vi "testing_camera_settings.vi"() -> ()   [LabVIEW 2015]
panel:
  out "Expected Rate":dbl
  out "millisecond timer value":u32
  out "imaq error":errorcluster
  out "dcam error":errorcluster {"code" format="%.0x"}
  out "Acquiring Frames":bool
  out "Frames Recorded":i32
  out "Display":T1(plugin-control)
  out "Current Stim Frames":i32
  out "H Width":i32
  out "V Width":i32
  out "Exposure":dbl
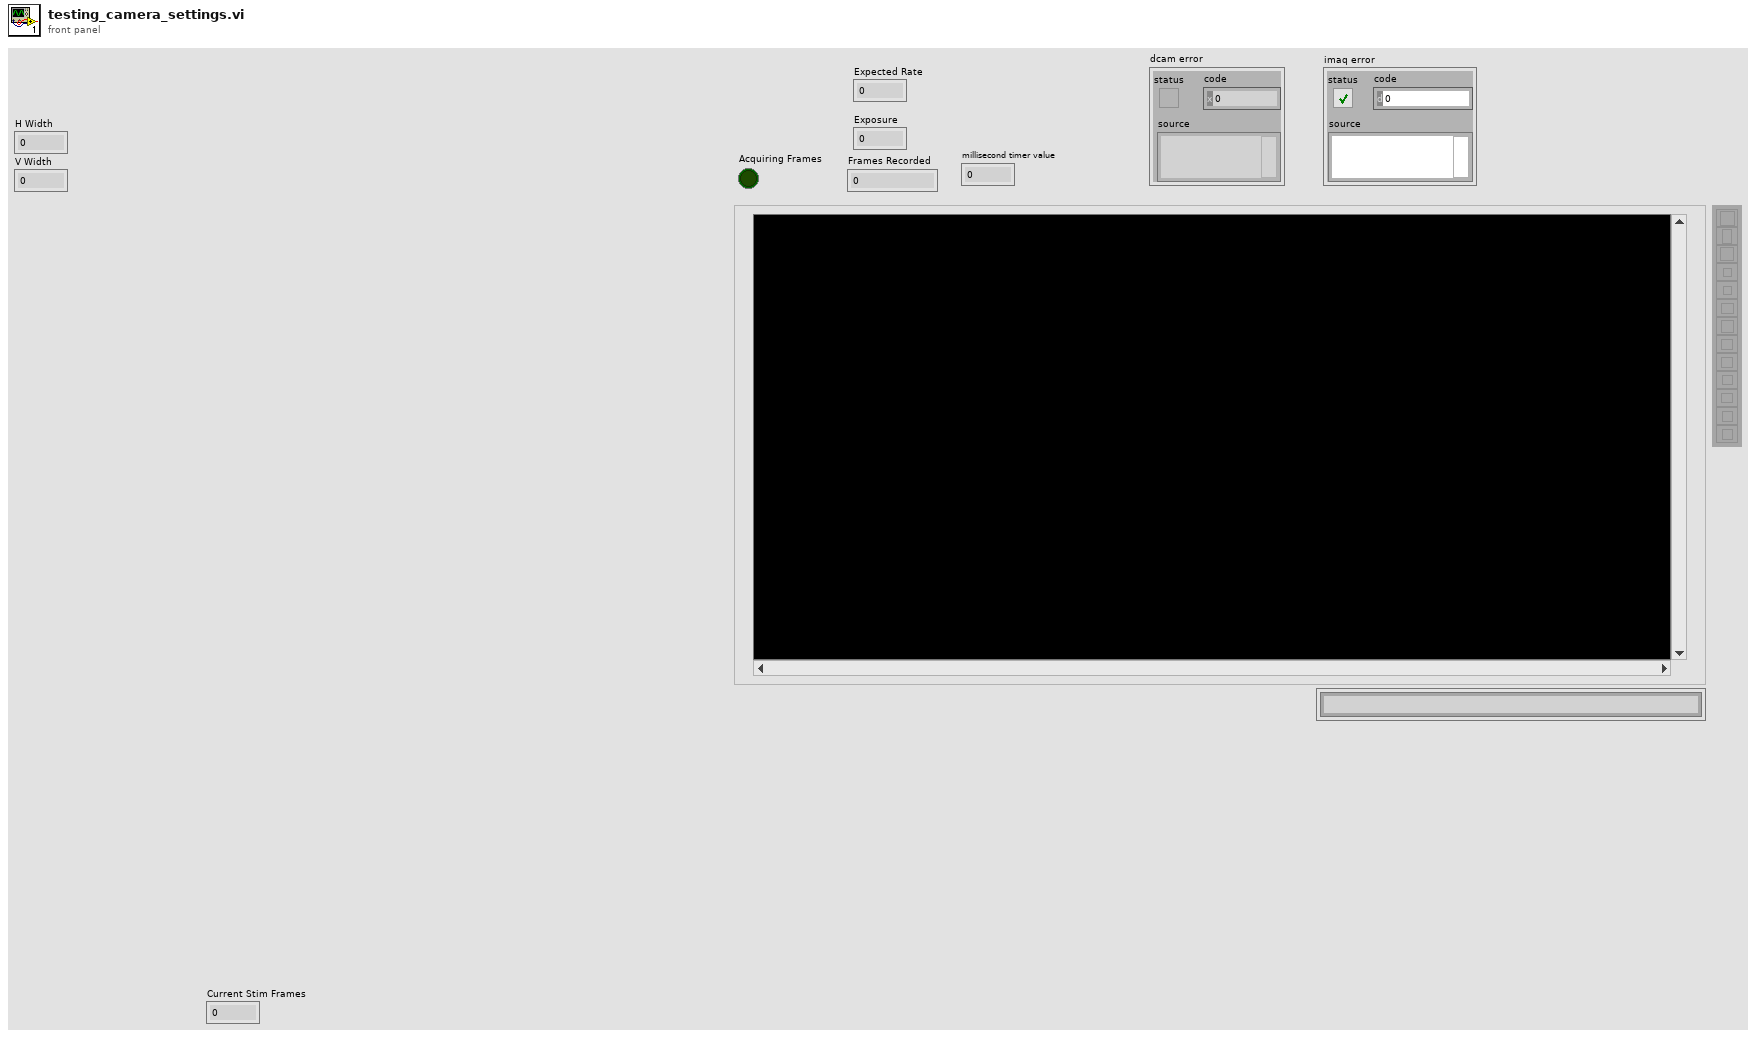
[diagram p1: front panel]
types:
  T1 = typedef "IMAQ Image.ctl" = refnum<image>
  T2 = cluster{"Mode":u32, "Polarity":u32, "Period":dbl, "Delay":dbl}
  T3 = typedef "Image Type" = u32
  T4 = cluster{"Value":i32, "Minimum":i32, "Maximum":i32, "Increment":i32}
  T5 = cluster{"height":u32, "width":u32, "datatype":u32}
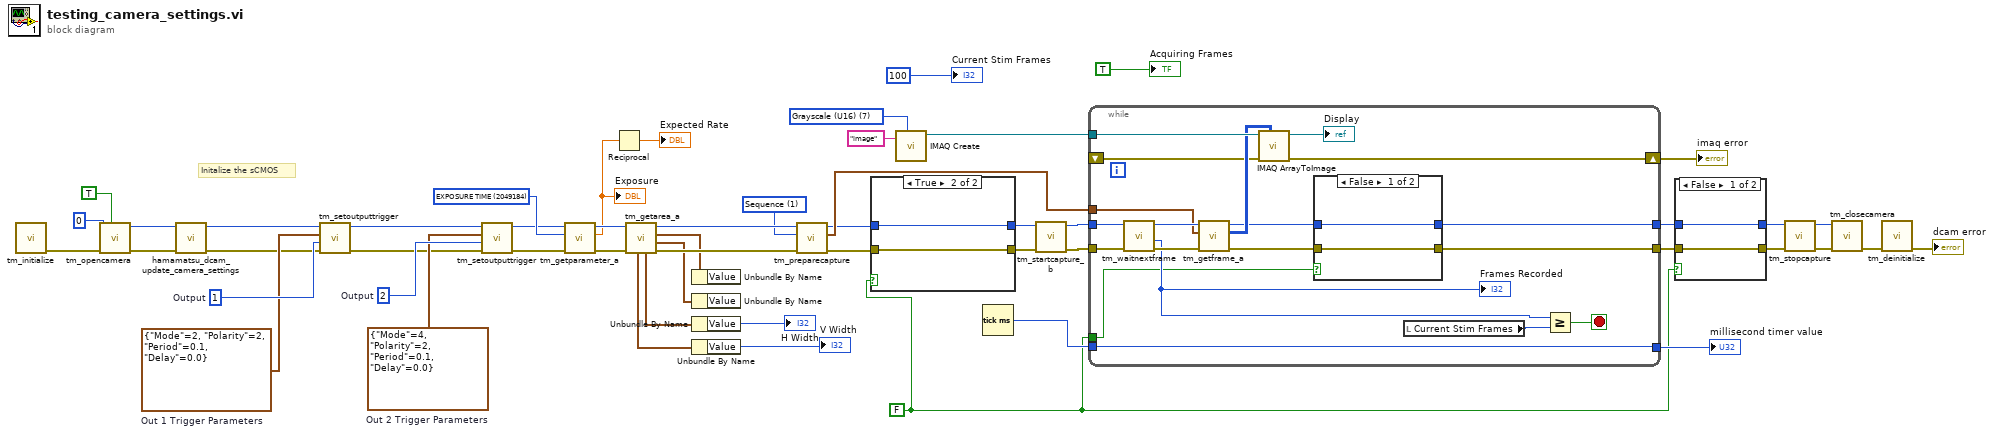
[diagram p0: block diagram]
diagram:
  w11 = FALSE ("Boolean")
  w22 = T2 {"Mode"=4, "Polarity"=2, "Period"=0.1, "Delay"=0.0}  # Out 2 Trigger Parameters
  w23 = T2 {"Mode"=2, "Polarity"=2, "Period"=0.1, "Delay"=0.0}  # Out 1 Trigger Parameters
  w24 = 2  # Output
  w25 = 1  # Output
  w36 = u32 2049184 items=["SENSOR MODE"=4212128, "CCD MODE"=4212384, "READOUT MODE"=4211872, "ACTIVE VIEW INDEX"=4343136, "BITS PER CHANNEL"=4342976, "IMAGE PIXEL TYPE"=4343296, "BINNING"=4215968, "EXPOSURE TIME"=2049184, "CONTRAST GAIN"=3163312, "CONTRAST OFFSET"=3163328, "LIGHT MODE"=2114720, "SENSITIVITY"=2114992, "PHOTON IMAGING MODE"=2115200, "HIGH DYNAMIC RANGE MODE"=3163360, "WHITE BALANCE"=3163568, "TEMPERATURE"=2115232, "TEMPERATURE TARGET"=2115264, "SENSOR COOLER FAN"=2115296, "LINEBUNDLE HEIGHT"=4212192, "MECHANICAL SHUTTER"=2115488, "BACK FOCUS POSITION"=8422304, "TRIGGER CONNECTOR"=1066432, "TRIGGER SOURCE"=1066144, "OUTPUT TRIGGER SOURCE"=1852576, "TRIGGER GLOBAL EXPOSURE"=2049680, "FIRST TRIGGER BEHAVIOR"=2049696, "CHANNEL SYNC"=1852352, "READOUT DIRECTION"=4211904, "PRE HSYNC COUNT"=1852704] ("Parameter")
  w42 = T3 7 items=["Grayscale (U8)", "Grayscale (I16)", "Grayscale (SGL)", "Complex (CSG)", "RGB (U32)", "HSL (U32)", "RGB (U64)", "Grayscale (U16)"] ("Image Type")
  w43 = 1 items=["Snap", "Sequence"] ("Capture mode")
  # "Initalize the sCMOS"
  n1 = call <userlib>:"tm_initialize.vi"() -> ("error out"=w39:errorcluster)  [unwired: 8 in, 3 out]
  n2 = call <userlib>:"tm_opencamera.vi"("Force Open"=TRUE, "error in (no error)"=w39, "Camera Index"=0) -> ("error out"=w26:errorcluster, "Handle out"=w27:u32)  [unwired: 6 in, 1 out]
  n3 = call "hamamatsu_dcam_update_camera_settings.vi"("error in (no error)"=w26, "Handle in"=w27) -> ("error out"=w16:errorcluster, "Handle out"=w17:u32)  [unwired: 6 in]
  n4 = call <userlib>:"tm_setoutputtrigger.vi"("error in (no error)"=w16, "Index"=w25, "Parameters"=w23, "Handle in"=w17) -> ("error out"=w21:errorcluster, "Handle out"=w20:u32)  [unwired: 6 in]
  n5 = call <userlib>:"tm_setoutputtrigger.vi"("error in (no error)"=w21, "Index"=w24, "Parameters"=w22, "Handle in"=w20) -> ("error out"=w19:errorcluster, "Handle out"=w18:u32)  [unwired: 6 in]
  n6 = call <userlib>:"tm_getparameter_a.vi"("error in (no error)"=w19, "Parameter"=w36, "Handle in"=w18) -> ("error out"=w31:errorcluster, "Value out"=w13:dbl, "Handle out"=w30:u32)  [unwired: 6 in]
  "Exposure" <- w13
  n7 = Reciprocal(x=w13) -> (1/x=→"Expected Rate":dbl)
  n8 = call <userlib>:"tm_getarea_a.vi"("error in (no error)"=w31, "Handle in"=w30) -> ("error out"=w49:errorcluster, "V Offset"=w34:T4, "H Offset"=w35:T4, "Handle out"=w50:u32, "H Width"=w33:T4, "V Width"=w32:T4)  [unwired: 4 in]
  n9 = Unbundle By Name(w35) -> ()  [unwired: 1 out]
  n10 = Unbundle By Name(w34) -> ()  [unwired: 1 out]
  n11 = Unbundle By Name(w33) -> ("Value"=→"H Width":i32)
  n12 = Unbundle By Name(w32) -> ("Value"=→"V Width":i32)
  n13 = call <userlib>:"tm_preparecapture.vi"("error in (no error)"=w49, "Capture mode"=w43, "Handle in"=w50) -> ("error out"=w5:errorcluster, "Buffer Info"=w53:T5, "Handle out"=w6:u32)  [unwired: 5 in, 1 out]
  n14 = case shown="True" w11 {
    tunnel: w6 -> [w55 w57]
    tunnel: w5 -> [w54 w56]
    tunnel: [w55 w57] -> w1
    tunnel: [w54 w56] -> w2
    frame False {
    }
    frame True {
    }
  }
  n15 = call "IMAQ Create"("Image Name"="image", "Image Type"=w42) -> ("New Image"=w52:T1)  [unwired: 3 in, 1 out]
  n16 = Tick Count (ms)() -> (millisecond timer value=w14:u32)
  n17 = call <userlib>:"tm_startcapture_b.vi"("error in (no error)"=w2, "Handle in"=w1) -> ("error out"=w3:errorcluster, "Handle out"=w4:u32)  [unwired: 8 in]
  n18 = while {
    tunnel: w3 -> [w74]
    tunnel: w53 -> [w73]
    tunnel: w4 -> [w72]
    tunnel: w52 -> [w69]
    shift-right: [w67] -> w44
    shift-left: _ -> [w66]
    tunnel: [w63] -> w15
    tunnel: w14 -> [w63]
    tunnel: w11 -> [w62]
    tunnel: [w59] -> w10
    tunnel: [w58] -> w9
    stop <- w70 stop-if-true
    n19 = call <userlib>:"tm_waitnextframe.vi"("error in (no error)"=w74, "Handle in"=w72) -> ("error out"=w76:errorcluster, "Frame Count"=w64:i32, "Handle out"=w75:u32)  [unwired: 6 in, 1 out]
    "Frames Recorded" <- w64
    n20 = call <userlib>:"tm_getframe_a.vi"("error in (no error)"=w76, "Buffer Info"=w73, "Handle in"=w75) -> ("error out"=w60:errorcluster, "Data 16"=w68:u16[][], "Handle out"=w61:u32)  [unwired: 4 in, 2 out]
    n21 = call "IMAQ ArrayToImage"("Image Pixels (U16)"=w68, "error in (no error)"=w66, "Image"=w69) -> ("error out"=w67:errorcluster, "Image Out"=→"Display":T1)  [unwired: 7 in]
    n22 = case shown="False" w62 {
      tunnel: w61 -> [w77 w80]
      tunnel: w60 -> [w78 w79]
      tunnel: [w78 w79] -> w59
      tunnel: [w77 w80] -> w58
      frame False {
      }
      frame True {
      }
    }
    n23 = local read "Current Stim Frames"() -> (w71:i32)
    n24 = Greater Or Equal?(x=w64, y=w71) -> (x >= y?=w70:bool)
  }
  "imaq error" <- w44
  "millisecond timer value" <- w15
  n25 = case shown="False" w11 {
    tunnel: w10 -> [w81 w83]
    tunnel: w9 -> [w82 w84]
    tunnel: [w82 w84] -> w8
    tunnel: [w81 w83] -> w7
    frame False {
    }
    frame True {
    }
  }
  n26 = call <userlib>:"tm_stopcapture.vi"("error in (no error)"=w7, "Handle in"=w8) -> ("error out"=w46:errorcluster, "Handle out"=w45:u32)  [unwired: 8 in]
  n27 = call <userlib>:"tm_closecamera.vi"("error in (no error)"=w46, "Handle in"=w45) -> ("error out"=w48:errorcluster)  [unwired: 9 in]
  n28 = call <userlib>:"tm_deinitialize.vi"("error in (no error)"=w48) -> ("error out"=→"dcam error":errorcluster)  [unwired: 10 in]
  "Current Stim Frames" <- 100 ("Current Stim Frames")
  "Acquiring Frames" <- TRUE
